vi "GFGTranslator.vi"(6 "boolean_ip":bool, 7 "Action":string, 8 "numeric_ip":dbl, 9 "string_ip":string="no. frames to acquire", 10 "GFG_var_name":string="no. frames to acquire", 11 "DataType":string) -> (0 "boolean_op":bool, 1 "numeric_op":dbl, 2 "string_op":string="no. frames to acquire", 3 "status":string, 4 "variant_op":variant, 5 "array_op":i16[][](array[numeric]))   [LabVIEW 2012]
doc: "SciScan 1.2 160622\nGFGTranslator 1.1 151001\n\nThis VI acts as an intermediate between a Python script and the LabVIEW SciScan application. Before using this VI make sure that the file path is correctly set to point to GFG_Core.ref file (situated in the SciScan project folder).\n\nAnother thing to note is that this VI should NOT be included in a project (i.e., needs to be run as a stand-alone VI), else could result in LabVIEW crashing"
uses:
  <vilib>/Utility/VariantDataType/Type.ctl
  <vilib>/vision/Image Controls.llb/IMAQ Image.ctl
  <vilib>/Utility/VariantDataType/VariantType.lvlib
  <vilib>/regexp/Match Regular Expression.xnode
panel:
  # "INPUTS"
  # "OUTPUTS"
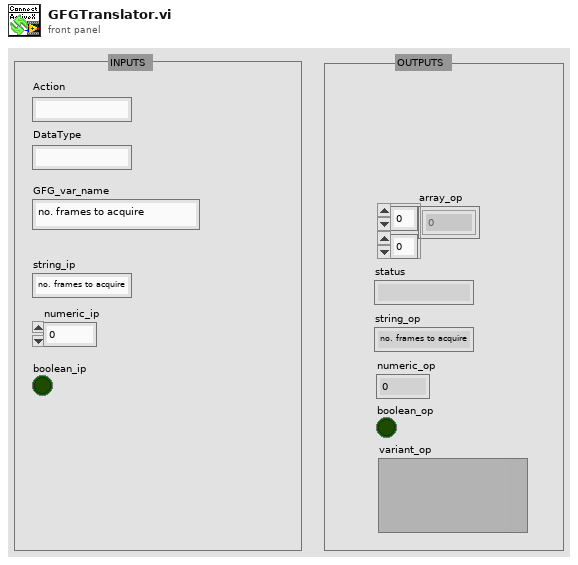
[diagram p1: front panel]
types:
  T1 = enum16{"open", "replace", "create", "open or create", "replace or create", "replace or create with confirmation"}
  T2 = typedef "VariantType.lvlib/Type.ctl" = enum8{"Invalid Type", "Void", "I8", "I16", "I32", "I64", "U8", "U16", "U32", "U64", "Single Float", "Double Float", "Extended Float", "Single Complex", "Double Complex", "Extended Complex", "Enum U8", "Enum U16", "Enum U32", "Enum U64", "Single Float With Unit", "Double Float With Unit", "Extended Float With Unit", "Single Complex with Unit", "Double Complex with Unit", "Extended Complex with Unit", "Boolean", "String", "Path", "Picture", "Tag", "Array", "Cluster", "Variant", "LV Variant", "Waveform", "Timestamp", "Digital Waveform", "Digital Data", "ExpressData", "Refnum", "External Data", "VI", "Poly VI", "LabVIEW Class Instance", "Fixed Point"}
  T3 = typedef "IMAQ Image.ctl" = refnum<image>
  T4 = cluster{"Channel 1 small":T3, "Channel 2 small":T3, "Channel 3 small":T3, "Channel 4 small":T3, "Channel 1 large":T3, "Channel 2 large":T3, "Channel 3 large":T3, "Channel 4 large":T3, "RGB overlay":T3, "ROI Image display":T3, "arb line scan display":T3, "Channel 5 large":T3}
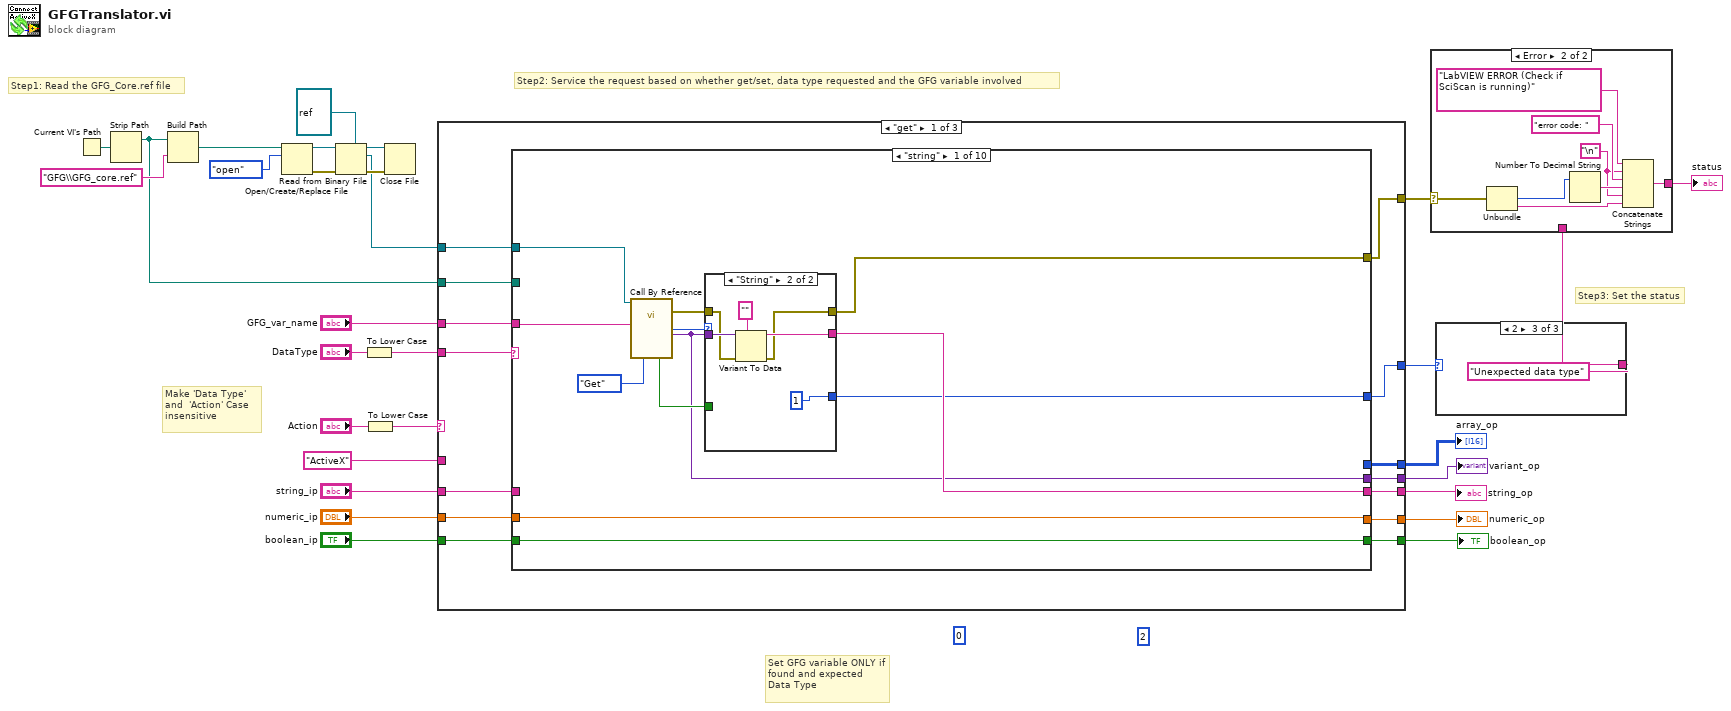
[diagram p0: block diagram]
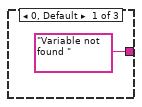
[diagram p3: hidden frame]
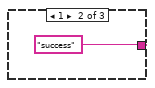
[diagram p4: hidden frame]
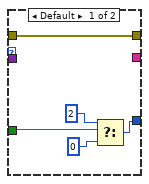
[diagram p5: hidden frame]
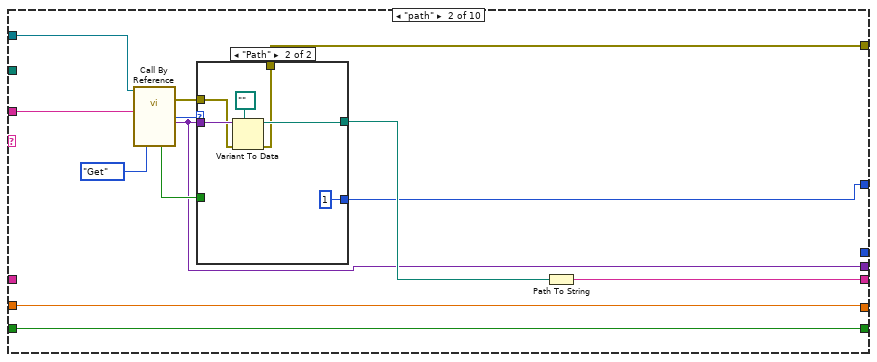
[diagram p6: hidden frame]
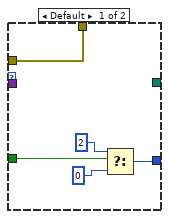
[diagram p7: hidden frame]
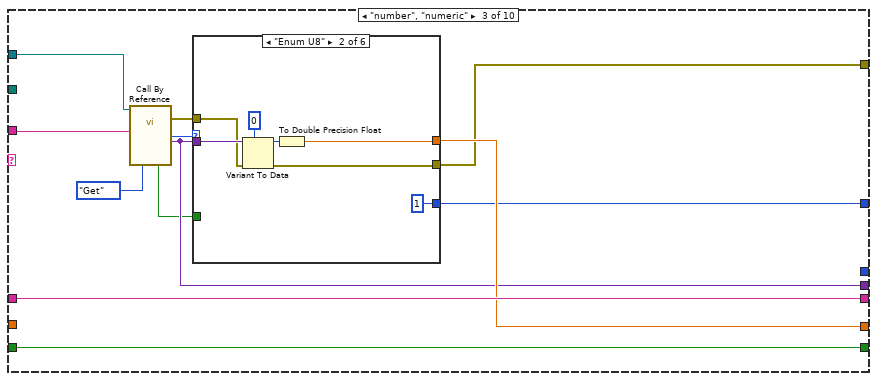
[diagram p8: hidden frame]
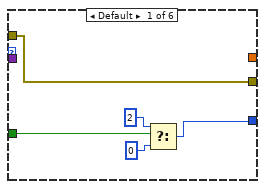
[diagram p9: hidden frame]
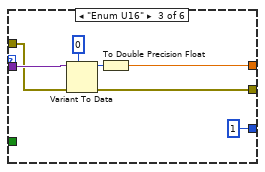
[diagram p10: hidden frame]
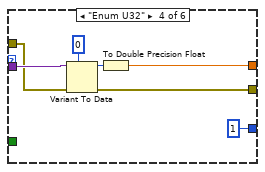
[diagram p11: hidden frame]
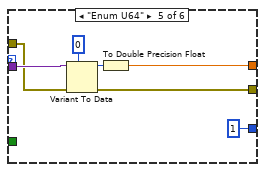
[diagram p12: hidden frame]
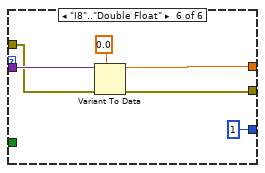
[diagram p13: hidden frame]
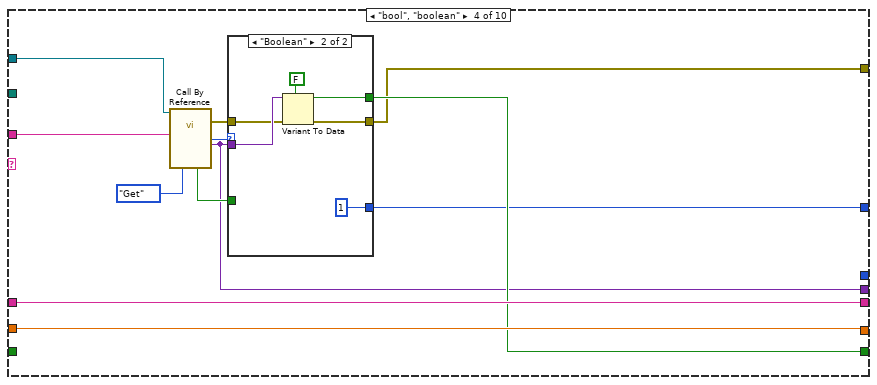
[diagram p14: hidden frame]
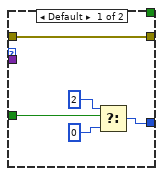
[diagram p15: hidden frame]
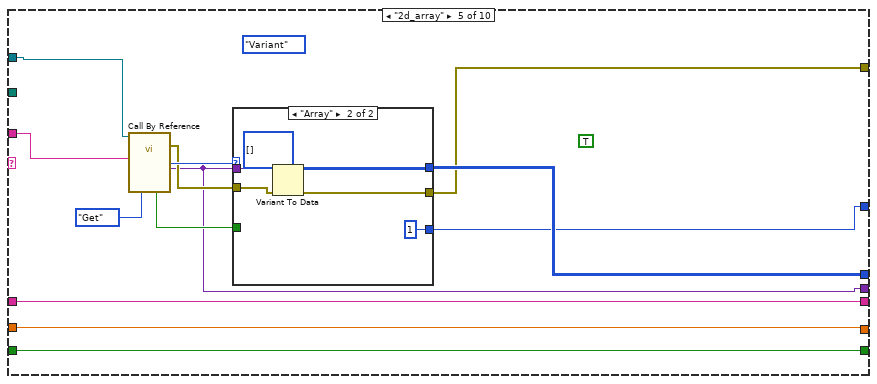
[diagram p16: hidden frame]
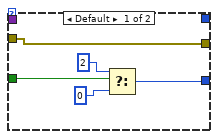
[diagram p17: hidden frame]
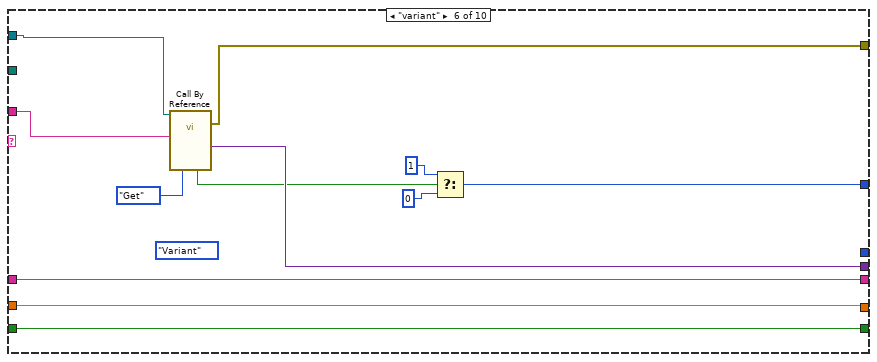
[diagram p18: hidden frame]
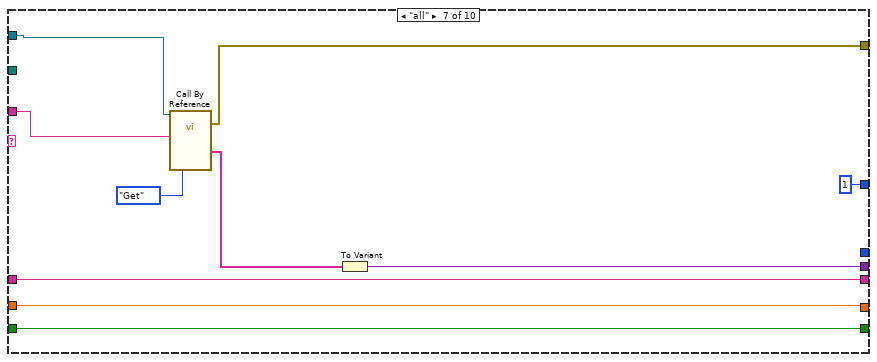
[diagram p19: hidden frame]
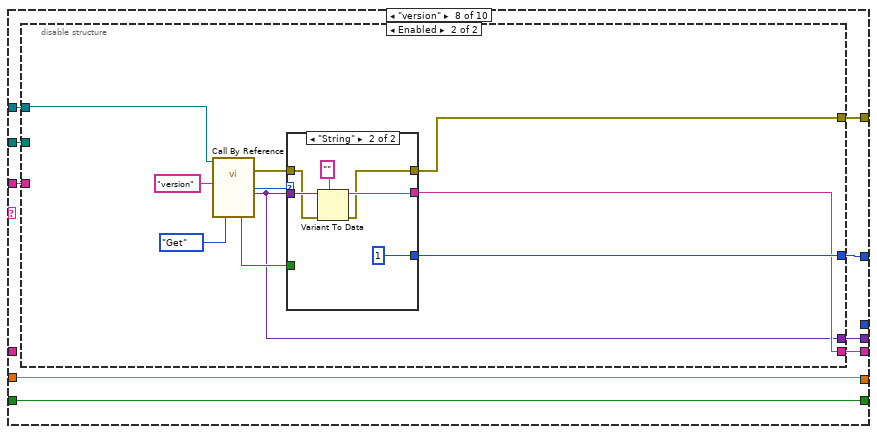
[diagram p20: hidden frame]
diagram:
  (unwired) 0
  (unwired) 2
  # "Set GFG variable ONLY if found and expected Data Type"
  # "Step3: Set the status"
  # "Step2: Service the request based on whether get/set, data type requested and the GFG variable involved"
  # "Step1: Read the GFG_Core.ref file"
  # "Make 'Data Type'\nand  'Action' Case\ninsensitive"
  n1 = Current VI's Path() -> (path=w10:path)
  n2 = Strip Path(path=w10) -> (stripped path=w7:path)  [unwired: 1 out]
  n3 = Build Path(base path=w7, name or relative path="GFG\\GFG_core.ref") -> (appended path=w8:path)
  n4 = Open/Create/Replace File(file path (use dialog)=w8, operation (0:open)=T1."open") -> (refnum out=w17:refnum<file>, error out=w18:errorcluster)  [unwired: 4 in, 1 out]
  n5 = Read from Binary File(5:refnum<vi> refnum ("type specifier VI Refnum (for type only)"), 8:w18, 11:w17) -> (0:w15:errorcluster, 2:w13:refnum<vi>, 3:w16:refnum<file>)  [unwired: 3 in, 1 out]
  n6 = To Lower Case(string="DataType") -> (all lower case string=w20:string)
  n7 = To Lower Case(string="Action") -> (all lower case string=w21:string)
  n8 = Close File(refnum=w16, error in=w15) -> ()  [unwired: 2 out]
  n9 = case shown="\"get\"" w21 {
    tunnel: w20 -> [w43 _ w578]
    tunnel: "GFG_var_name" -> [w42 _ w587]
    tunnel: [w41 w575 w585] -> w3
    tunnel: w13 -> [w40 _ w584]
    tunnel: "string_ip" -> [w38 w575 w586]
    tunnel: "ActiveX" ("Source VI") -> [_ _ w583]
    tunnel: "numeric_ip" -> [w37 w574 w582]
    tunnel: "boolean_ip" -> [w36 w573 w581]
    tunnel: [w39 w574 w580] -> w2
    tunnel: [w35 w573 w579] -> w22
    tunnel: [w34 _ _] -> w12
    tunnel: [w33 _ _] -> w11
    tunnel: w7 -> [w32 _ _]
    tunnel: [w31 errorcluster {"status"=TRUE, "code"=0, "source"="Undefined command received from ActiveX client"} ("error out") w577] -> w6
    tunnel: [w30 0 w576] -> w1
    frame "get" {
      n10 = case shown="\"string\"" w43 {
        tunnel: w42 -> [w51 w74 w98 w149 w173 w197 w207 w215 w527 _]
        tunnel: [w49 w79 w102 w152 w176 w199 w209 w216 w542 w570] -> w41
        tunnel: w40 -> [w50 w73 w97 w148 w172 w196 w204 w213 w537 _]
        tunnel: [w55 w78 w96 w153 w177 w200 w210 w219 w543 w569] -> w39
        tunnel: w38 -> [_ _ w102 w152 w176 w199 w209 _ w542 w570]
        tunnel: w37 -> [w55 w78 _ w153 w177 w200 w210 w219 w543 w569]
        tunnel: w36 -> [w54 w77 w101 _ w171 w195 w206 w218 w541 w568]
        tunnel: [w54 w77 w101 w147 w171 w195 w206 w218 w541 w568] -> w35
        tunnel: [_ _ _ _ w170 _ _ _ w540 _] -> w34
        tunnel: [w44 w67 w95 w142 w165 w194 w205 w211 w525 _] -> w33
        tunnel: w32 -> [_ _ _ _ _ _ _ w217 _ _]
        tunnel: [w47 w71 w94 w145 w168 w193 w203 w214 w529 errorcluster {"status"=TRUE, "code"=0, "source"="Undefined data Type"} ("error out")] -> w31
        tunnel: [w45 w68 w91 w143 w166 w189 1 w212 w528 2] -> w30
        frame "string" {
          n11 = call-by-ref "?"(reference=w50, "Variable Name in"=w51, "Action"=enum16{"Init", "Set", "Get"}."Get") -> (error out=w48:errorcluster, "Found/Replaced"=w46:bool, "Data Type Out"=w53:T2, "Variant Out"=w44:variant)  [unwired: 12 in, 5 out]
          n12 = case shown="\"String\"" w53 {
            tunnel: w44 -> [_ w66]
            tunnel: [_ w65] -> w49
            tunnel: w48 -> [w60 w63]
            tunnel: [w60 w62] -> w47
            tunnel: w46 -> [w58 _]
            tunnel: [w57 1] -> w45
            frame Default {
              n13 = Select(t=2, s=w58, f=0) -> (s? t:f=w57:i32)
            }
            frame "String" {
              n14 = Variant To Data(error in=w63, type="" ("string_ip"), Variant=w66) -> (data=w65:string, error out=w62:errorcluster)
            }
          }
        }
        frame "path" {
          n15 = call-by-ref "?"(reference=w73, "Variable Name in"=w74, "Action"=enum16{"Init", "Set", "Get"}."Get") -> (error out=w70:errorcluster, "Found/Replaced"=w69:bool, "Data Type Out"=w76:T2, "Variant Out"=w67:variant)  [unwired: 12 in, 5 out]
          n16 = case shown="\"Path\"" w76 {
            tunnel: w67 -> [_ w90]
            tunnel: [_ w89] -> w72
            tunnel: [w84 w87] -> w71
            tunnel: w70 -> [w84 w86]
            tunnel: w69 -> [w81 _]
            tunnel: [w80 1] -> w68
            frame Default {
              n17 = Select(t=2, s=w81, f=0) -> (s? t:f=w80:i32)
            }
            frame "Path" {
              n18 = Variant To Data(error in=w86, type=path "" ("Path"), Variant=w90) -> (data=w89:path, error out=w87:errorcluster)
            }
          }
          n19 = Path To String(path=w72) -> (string=w79:string)
        }
        frame "number", "numeric" {
          n20 = call-by-ref "?"(reference=w97, "Variable Name in"=w98, "Action"=enum16{"Init", "Set", "Get"}."Get") -> (error out=w93:errorcluster, "Found/Replaced"=w92:bool, "Data Type Out"=w100:T2, "Variant Out"=w95:variant)  [unwired: 12 in, 5 out]
          n21 = case shown="\"Enum U8\"" w100 {
            tunnel: w95 -> [_ w112 w119 w126 w133 w140]
            tunnel: [_ w111 w118 w125 w132 w139] -> w96
            tunnel: [w107 w109 w116 w123 w131 w138] -> w94
            tunnel: w93 -> [w107 w110 w117 w124 w130 w137]
            tunnel: w92 -> [w104 _ _ _ _ _]
            tunnel: [w103 1 1 1 1 1] -> w91
            frame Default {
              n22 = Select(t=2, s=w104, f=0) -> (s? t:f=w103:i32)
            }
            frame "Enum U8" {
              n23 = Variant To Data(error in=w110, type=u8 0 ("numeric_ip"), Variant=w112) -> (data=w113:u8, error out=w109:errorcluster)
              n24 = To Double Precision Float(number=w113) -> (double precision float=w111:dbl)
            }
            frame "Enum U16" {
              n25 = Variant To Data(error in=w117, type=u16 0 ("numeric_ip"), Variant=w119) -> (data=w120:u16, error out=w116:errorcluster)
              n26 = To Double Precision Float(number=w120) -> (double precision float=w118:dbl)
            }
            frame "Enum U32" {
              n27 = Variant To Data(error in=w124, type=u32 0 ("numeric_ip"), Variant=w126) -> (data=w127:u32, error out=w123:errorcluster)
              n28 = To Double Precision Float(number=w127) -> (double precision float=w125:dbl)
            }
            frame "Enum U64" {
              n29 = Variant To Data(error in=w130, type=u64 0 ("numeric_ip"), Variant=w133) -> (data=w134:u64, error out=w131:errorcluster)
              n30 = To Double Precision Float(number=w134) -> (double precision float=w132:dbl)
            }
            frame "I8".."Double Float" {
              n31 = Variant To Data(error in=w137, type=0.0 ("numeric_ip"), Variant=w140) -> (data=w139:dbl, error out=w138:errorcluster)
            }
          }
        }
        frame "bool", "boolean" {
          n32 = call-by-ref "?"(reference=w148, "Variable Name in"=w149, "Action"=enum16{"Init", "Set", "Get"}."Get") -> (error out=w146:errorcluster, "Found/Replaced"=w144:bool, "Data Type Out"=w151:T2, "Variant Out"=w142:variant)  [unwired: 12 in, 5 out]
          n33 = case shown="\"Boolean\"" w151 {
            tunnel: w142 -> [_ w164]
            tunnel: [_ w162] -> w147
            tunnel: w146 -> [w158 w161]
            tunnel: [w158 w160] -> w145
            tunnel: w144 -> [w157 _]
            tunnel: [w154 1] -> w143
            frame Default {
              n34 = Select(t=2, s=w157, f=0) -> (s? t:f=w154:i32)
            }
            frame "Boolean" {
              n35 = Variant To Data(error in=w161, type=FALSE, Variant=w164) -> (data=w162:bool, error out=w160:errorcluster)
            }
          }
        }
        frame "2d_array" {
          (unwired) TRUE ("Found/Replaced")
          (unwired) Type."Variant" ("Data Type Out")
          n36 = call-by-ref "?"(reference=w172, "Variable Name in"=w173, "Action"=enum16{"Init", "Set", "Get"}."Get") -> (error out=w169:errorcluster, "Found/Replaced"=w167:bool, "Data Type Out"=w175:T2, "Variant Out"=w165:variant)  [unwired: 12 in, 5 out]
          n37 = case shown="\"Array\"" w175 {
            tunnel: w165 -> [_ w188]
            tunnel: [_ w187] -> w170
            tunnel: w169 -> [w182 w185]
            tunnel: [w182 w184] -> w168
            tunnel: w167 -> [w179 _]
            tunnel: [w178 1] -> w166
            frame Default {
              n38 = Select(t=2, s=w179, f=0) -> (s? t:f=w178:i32)
            }
            frame "Array" {
              n39 = Variant To Data(error in=w185, type=i16[][] [], Variant=w188) -> (data=w187:i16[][], error out=w184:errorcluster)
            }
          }
        }
        frame "variant" {
          (unwired) Type."Variant" ("Data Type Out")
          n40 = call-by-ref "?"(reference=w196, "Variable Name in"=w197, "Action"=enum16{"Init", "Set", "Get"}."Get") -> (error out=w193:errorcluster, "Found/Replaced"=w190:bool, "Variant Out"=w194:variant)  [unwired: 12 in, 6 out]
          n41 = Select(t=1, s=w190, f=0) -> (s? t:f=w189:i32)
        }
        frame "all" {
          n42 = call-by-ref "?"(reference=w204, "Variable Name in"=w207, "Action"=enum16{"Init", "Set", "Get"}."Get") -> (error out=w203:errorcluster, "All Variable Names Out"=w202:string[])  [unwired: 12 in, 7 out]
          n43 = To Variant(anything=w202) -> (Variant=w205:variant)
        }
        frame "version" {
          n44 = disable-structure shown="Enabled" {
            disable-tunnel: w217 -> [w227 _]
            disable-tunnel: [w226 w505] -> w216
            disable-tunnel: w215 -> [w224 _]
            disable-tunnel: [w223 w507] -> w214
            disable-tunnel: w213 -> [w221 w509]
            disable-tunnel: [w220 w506] -> w212
            disable-tunnel: [_ w504] -> w211
            frame Disabled {
              n45 = To Lower Case(string=w224) -> (all lower case string=w228:string)
              n46 = xnode "Match Regular Expression"("input string"=w228, "regular expression"=".lvproj|.vi") -> ("before match"=w225:string, "error out"=w222:errorcluster)  [unwired: 4 in, 3 out]
              n47 = case shown="Default" w225 {
                selector: w225 -> [_ w357 _]
                tunnel: w227 -> [w344 _ _]
                tunnel: [w349 w362 w499] -> w226
                tunnel: [w348 w356 w497] -> w223
                tunnel: w222 -> [w347 w355 w496]
                tunnel: w221 -> [_ _ _]
                tunnel: [1 w354 1] -> w220
                frame "sci_scan", "sciscan" {
                  n48 = Build Path(base path=w344, name or relative path="Sci_Scan.lvproj") -> (appended path=w342:path)
                  n49 = invoke class="App" method="Project.Open"(error in=w347, "Path"=w342) -> (error out=w345:errorcluster, "Project:Open"=w346:refnum<vi>)  [unwired: 2 in, 2 out]
                  n50 = property class="Project"(reference=w346, error in=w345) -> (reference out=w352:refnum<vi>, error out=w353:errorcluster, "Description"=w351:string)
                  n51 = Close Reference(reference=w352, error in (no error)=w353) -> (error out=w348:errorcluster)
                  n52 = Match Pattern(string=w351, regular expression="[\\n,\\r]") -> (before substring=w349:string)  [unwired: 1 in, 3 out]
                }
                frame Default {
                  n53 = call "get all VIs in SciScan directory.vi"() -> ("All Files in Dir"=w358:path[])  [unwired: 11 in]
                  n54 = for {
                    tunnel: w358 -> [w367] mode=indexing
                    tunnel: [w364] -> w359 mode=indexing
                    n55 = Strip Path(path=w367) -> (name=w365:string)  [unwired: 1 out]
                    n56 = To Lower Case(string=w365) -> (all lower case string=w366:string)
                    n57 = xnode "Match Regular Expression"("input string"=w366, "regular expression"=".lvproj|.vi") -> ("before match"=w364:string)  [unwired: 4 in, 4 out]
                  }
                  n58 = Search 1D Array(1D array=w359, element=w357) -> (index of element=w361:i32)  [unwired: 1 in]
                  n59 = Greater Or Equal To 0?(x=w361) -> (x >= 0?=w360:bool)
                  n60 = case shown="False" w360 {
                    tunnel: ["The specified project/VI name not found" ("Description") w493] -> w362
                    tunnel: w361 -> [_ w490]
                    tunnel: w358 -> [_ w486]
                    tunnel: [w480 w485] -> w356
                    tunnel: w355 -> [w480 w484]
                    tunnel: [0 1] -> w354
                    frame False {
                    }
                    frame True {
                      n61 = Index Array(array=w486, index=w490) -> (element=w489:path)
                      n62 = Open VI Reference(vi path=w489, error in (no error)=w484) -> (vi reference=w492:refnum<vi>, error out=w483:errorcluster)  [unwired: 4 in]
                      n63 = property class="VI"(reference=w492, error in=w483) -> (reference out=w487:refnum<vi>, error out=w488:errorcluster, "Description"=w491:string)
                      n64 = Match Pattern(string=w491, regular expression="[\\n,\\r]") -> (before substring=w493:string)  [unwired: 1 in, 3 out]
                      n65 = Close Reference(reference=w487, error in (no error)=w488) -> (error out=w485:errorcluster)
                    }
                  }
                }
                frame "gfgtranslator" {
                  n66 = control-ref of="This VI"() -> (w498:refnum<vi>)
                  n67 = property class="VI"(reference=w498, error in=w496) -> (reference out=w502:refnum<vi>, error out=w503:errorcluster, "Description"=w501:string)
                  n68 = Close Reference(reference=w502, error in (no error)=w503) -> (error out=w497:errorcluster)
                  n69 = Match Pattern(string=w501, regular expression="[\\n,\\r]") -> (before substring=w499:string)  [unwired: 1 in, 3 out]
                }
              }
            }
            frame Enabled {
              n70 = call-by-ref "?"(reference=w509, "Variable Name in"="version", "Action"=enum16{"Init", "Set", "Get"}."Get") -> (error out=w511:errorcluster, "Found/Replaced"=w510:bool, "Data Type Out"=w513:T2, "Variant Out"=w504:variant)  [unwired: 12 in, 5 out]
              n71 = case shown="\"String\"" w513 {
                tunnel: w504 -> [_ w524]
                tunnel: [_ w523] -> w505
                tunnel: w511 -> [w518 w521]
                tunnel: [w518 w520] -> w507
                tunnel: w510 -> [w516 _]
                tunnel: [w515 1] -> w506
                frame Default {
                  n72 = Select(t=2, s=w516, f=0) -> (s? t:f=w515:i32)
                }
                frame "String" {
                  n73 = Variant To Data(error in=w521, type="" ("string_ip"), Variant=w524) -> (data=w523:string, error out=w520:errorcluster)
                }
              }
            }
          }
        }
        frame "image" {
          w535 = T4 {"Channel 1 small"=refnum, "Channel 2 small"=refnum, "Channel 3 small"=refnum, "Channel 4 small"=refnum, "Channel 1 large"=refnum, "Channel 2 large"=refnum, "Channel 3 large"=refnum, "Channel 4 large"=refnum, "RGB overlay"=refnum, "ROI Image display"=refnum, "arb line scan display"=refnum, "Channel 5 large"=refnum}  # output cluster
          n74 = call-by-ref "?"(reference=w537, "Variable Name in"="ImageRefCluster", "Action"=enum16{"Init", "Set", "Get"}."Get") -> (reference out=w526:refnum<vi>, error out=w530:errorcluster, "Variant Out"=w525:variant)  [unwired: 12 in, 6 out]
          n75 = Variant To Data(error in=w530, type=w535, Variant=w525) -> (data=w534:T4, error out=w533:errorcluster)
          n76 = Cluster To Array(cluster=w534) -> (array=w536:T3[])
          n77 = case shown="No Error" w533 {
            selector: w533 -> [w546 w555]
            tunnel: w536 -> [w549 _]
            tunnel: w527 -> [w548 _]
            tunnel: [w547 _] -> w531
            tunnel: [w545 _] -> w532
            tunnel: [w544 w555] -> w529
            frame No Error {
              n78 = for {
                tunnel: w549 -> [w550] mode=indexing
                tunnel: w548 -> [w553]
                tunnel: [w552] -> w547
                tunnel: [w550] -> w545
                tunnel: w546 -> [_]
                tunnel: [w551] -> w544
                stop <- w552 stop-if-true
                n79 = call "IMAQ GetImageInfo"("Image"=w550) -> ("error out"=w551:errorcluster, "Image Name"=w554:string)  [unwired: 3 in, 6 out]
                n80 = Equal?(x=w554, y=w553) -> (x = y?=w552:bool)
              }
            }
            frame Error {
            }
          }
          n81 = case shown="False" w531 {
            tunnel: [_ w565] -> w540
            tunnel: w532 -> [_ w564]
            tunnel: [w556 1] -> w528
            tunnel: w527 -> [w561 _]
            tunnel: w526 -> [w560 _]
            frame False {
              # "The variable has not been found in the ImageRefCluster.\nCheck if the variable is present in the GFG and report error accordingly"
              n82 = call-by-ref "?"(reference=w560, "Variable Name in"=w561, "Action"=enum16{"Init", "Set", "Get"}."Get") -> ("Found/Replaced"=w557:bool)  [unwired: 12 in, 8 out]
              n83 = Select(t=2, s=w557, f=0) -> (s? t:f=w556:i32)
            }
            frame True {
              n84 = call "IMAQ ImageToArray"("Image"=w564) -> ("Image Pixels (I16)"=w565:i16[][])  [unwired: 3 in, 4 out]
            }
          }
        }
        frame Default {
        }
      }
    }
    frame Default {
    }
    frame "set" {
      n85 = case shown="\"booleanref\"" w578 {
        tunnel: w587 -> [w592 w641 w673 w718 w752 _]
        tunnel: w586 -> [w600 w648 w680 w725 w765 w804]
        tunnel: [w600 w648 w680 w725 w765 w804] -> w585
        tunnel: w584 -> [w596 w643 w676 w721 w751 _]
        tunnel: w583 -> [w599 _ w668 w726 _ _]
        tunnel: w582 -> [w598 w645 w679 w723 w764 w805]
        tunnel: w581 -> [w597 w646 w678 w724 w750 w806]
        tunnel: [w598 w645 w679 w723 w764 w805] -> w580
        tunnel: [w597 w646 w678 w724 w750 w806] -> w579
        tunnel: [w591 w638 w671 w716 w749 errorcluster {"status"=TRUE, "code"=0, "source"="Undefined data type received from ActiveX client"} ("error out")] -> w577
        tunnel: [w588 w636 w669 w714 w747 2 ("f")] -> w576
        frame "string" {
          # "Check if GFG variable exists"
          # "Set GFG variable ONLY if found and expected Data Type"
          n86 = call-by-ref "?"(reference=w596, "Variable Name in"=w592, "Action"=enum16{"Init", "Set", "Get", "Clear"}."Get") -> (reference out=w595:refnum<vi>, error out=w594:errorcluster, "Found/Replaced"=w590:bool, "Data Type Out"=w589:T2)  [unwired: 12 in, 5 out]
          n87 = case shown="True" w590 {
            tunnel: w600 -> [w604 w625]
            tunnel: w599 -> [w602 w624]
            tunnel: w595 -> [w603 w623]
            tunnel: w594 -> [w605 w622]
            tunnel: w592 -> [w606 w621]
            tunnel: [w601 w620] -> w591
            tunnel: w589 -> [_ w619]
            tunnel: [w607 w618] -> w588
            frame False {
              n88 = case shown="\"SetAbsXYZ\", \"SetVirtXYZ\"" w606 {
                selector: w606 -> [_ w615]
                tunnel: [0 1] -> w607
                tunnel: w605 -> [w608 w612]
                tunnel: w604 -> [_ w614]
                tunnel: w603 -> [_ w611]
                tunnel: w602 -> [_ w613]
                tunnel: [w608 w610] -> w601
                frame Default {
                }
                frame "SetAbsXYZ", "SetVirtXYZ" {
                  n89 = call-by-ref "?"(reference=w611, error in=w612, "Variable Name in"=w615, "Variant in"=w614, "Source VI"=w613, "Action"=enum16{"Init", "Set", "Get", "Clear"}."Set") -> (error out=w610:errorcluster)  [unwired: 9 in, 8 out]
                }
              }
            }
            frame True {
              n90 = case shown="\"String\"" w619 {
                tunnel: w625 -> [_ w635]
                tunnel: w624 -> [_ w634]
                tunnel: w623 -> [_ w633]
                tunnel: w622 -> [w627 w632]
                tunnel: w621 -> [_ w631]
                tunnel: [w627 w630] -> w620
                tunnel: [2 1] -> w618
                frame Default {
                }
                frame "String" {
                  n91 = call-by-ref "?"(reference=w633, error in=w632, "Variable Name in"=w631, "Variant in"=w635, "Source VI"=w634, "Action"=enum16{"Init", "Set", "Get", "Clear"}."Set") -> (error out=w630:errorcluster)  [unwired: 9 in, 8 out]
                }
              }
            }
          }
        }
        frame "path" {
          # "Set GFG variable ONLY if found and expected Data Type"
          # "Check if GFG variable exists"
          n92 = call-by-ref "?"(reference=w643, "Variable Name in"=w641, "Action"=enum16{"Init", "Set", "Get", "Clear"}."Get") -> (reference out=w642:refnum<vi>, error out=w639:errorcluster, "Found/Replaced"=w640:bool, "Data Type Out"=w637:T2)  [unwired: 12 in, 5 out]
          n93 = String To Path(string=w648) -> (path=w647:path)
          n94 = case shown="True" w640 {
            selector: w640 -> [_ w653]
            tunnel: w647 -> [_ w658]
            tunnel: w642 -> [_ w657]
            tunnel: w641 -> [_ w656]
            tunnel: w639 -> [w650 w655]
            tunnel: [w650 w654] -> w638
            tunnel: w637 -> [_ w652]
            tunnel: [0 w651] -> w636
            frame False {
            }
            frame True {
              n95 = case shown="\"Path\"" w652 {
                tunnel: w658 -> [_ w667]
                tunnel: w657 -> [_ w666]
                tunnel: w656 -> [_ w665]
                tunnel: w655 -> [w660 w664]
                tunnel: [w660 w663] -> w654
                tunnel: w653 -> [_ _]
                tunnel: [2 1] -> w651
                frame Default {
                }
                frame "Path" {
                  n96 = call-by-ref "?"(reference=w666, error in=w664, "Variable Name in"=w665, "Variant in"=w667, "Action"=enum16{"Init", "Set", "Get", "Clear"}."Set") -> (error out=w663:errorcluster)  [unwired: 10 in, 8 out]
                }
              }
            }
          }
        }
        frame "number", "numeric" {
          # "Set GFG variable ONLY if found and expected Data Type"
          # "Check if GFG variable exists"
          n97 = call-by-ref "?"(reference=w676, "Variable Name in"=w673, "Action"=enum16{"Init", "Set", "Get", "Clear"}."Get") -> (reference out=w675:refnum<vi>, error out=w674:errorcluster, "Found/Replaced"=w672:bool, "Data Type Out"=w670:T2)  [unwired: 12 in, 5 out]
          n98 = case shown="False" w672 {
            tunnel: w679 -> [w684 w704]
            tunnel: w675 -> [w686 w703]
            tunnel: w674 -> [w685 w702]
            tunnel: w673 -> [w681 w701]
            tunnel: [w682 w700] -> w671
            tunnel: w670 -> [_ w699]
            tunnel: [w687 w698] -> w669
            tunnel: w668 -> [w683 _]
            frame False {
              n99 = case shown="\"absX\", \"absY\", \"absZ\"" w681 {
                selector: w681 -> [_ w693]
                tunnel: [0 1] -> w687
                tunnel: w686 -> [_ w695]
                tunnel: w685 -> [w689 w694]
                tunnel: w684 -> [_ w692]
                tunnel: w683 -> [_ w691]
                tunnel: [w689 w690] -> w682
                frame "False", Default {
                }
                frame "absX", "absY", "absZ" {
                  n100 = call-by-ref "?"(reference=w695, error in=w694, "Variable Name in"=w693, "Variant in"=w692, "Source VI"=w691, "Action"=enum16{"Init", "Set", "Get", "Clear"}."Set") -> (error out=w690:errorcluster)  [unwired: 9 in, 8 out]
                }
              }
            }
            frame True {
              n101 = case shown="\"I8\"..\"Double Float\", \"Enum U8\"..\"Enum U64\"" w699 {
                tunnel: w704 -> [_ w713]
                tunnel: w703 -> [_ w712]
                tunnel: w702 -> [w705 w711]
                tunnel: w701 -> [_ w710]
                tunnel: [w705 w709] -> w700
                tunnel: [2 1] -> w698
                frame Default {
                }
                frame "I8".."Double Float", "Enum U8".."Enum U64" {
                  n102 = call-by-ref "?"(reference=w712, error in=w711, "Variable Name in"=w710, "Variant in"=w713, "Action"=enum16{"Init", "Set", "Get", "Clear"}."Set") -> (error out=w709:errorcluster)  [unwired: 10 in, 8 out]
                }
              }
            }
          }
        }
        frame "bool", "boolean" {
          # "Set GFG variable ONLY if found and expected Data Type"
          # "Check if GFG variable exists"
          n103 = call-by-ref "?"(reference=w721, "Variable Name in"=w718, "Action"=enum16{"Init", "Set", "Get", "Clear"}."Get") -> (reference out=w720:refnum<vi>, error out=w719:errorcluster, "Found/Replaced"=w717:bool, "Data Type Out"=w715:T2)  [unwired: 12 in, 5 out]
          n104 = case shown="False" w717 {
            tunnel: w726 -> [_ w736]
            tunnel: w724 -> [_ w735]
            tunnel: w720 -> [_ w734]
            tunnel: w719 -> [w728 w733]
            tunnel: w718 -> [_ w732]
            tunnel: [w728 w731] -> w716
            tunnel: w715 -> [_ w730]
            tunnel: [0 w729] -> w714
            frame False {
            }
            frame True {
              n105 = case shown="\"Boolean\"" w730 {
                tunnel: w736 -> [_ w746]
                tunnel: w735 -> [_ w745]
                tunnel: w734 -> [_ w744]
                tunnel: w733 -> [w738 w743]
                tunnel: w732 -> [_ w742]
                tunnel: [w738 w741] -> w731
                tunnel: [2 1] -> w729
                frame Default {
                }
                frame "Boolean" {
                  n106 = call-by-ref "?"(reference=w744, error in=w743, "Variable Name in"=w742, "Variant in"=w745, "Source VI"=w746, "Action"=enum16{"Init", "Set", "Get", "Clear"}."Set") -> (error out=w741:errorcluster)  [unwired: 9 in, 8 out]
                }
              }
            }
          }
        }
        frame "booleanref" {
          w757 = ".CtrlRef" ("string")
          # "Add a .CtrlRef"
          # "Set the Control ONLY if found, and the reference type is a 'Boolean Refnum'"
          # "Check if GFG variable exists"
          n107 = Search and Replace String(replace all?=TRUE ("replace all? (F)"), input string=w752, search string="[\\t \\r \\n \\s]+", replace string="." ("replace string (\"\")")) -> (result string=w756:string)  [unwired: 4 in, 3 out]
          n108 = Match Pattern(string=w756, regular expression=w757) -> (offset past match=w758:i32)  [unwired: 1 in, 3 out]
          n109 = case shown="-1" w758 {
            tunnel: [w798 w801] -> w760
            tunnel: w756 -> [w798 w800]
            tunnel: w757 -> [_ w799]
            frame 0, Default {
            }
            frame -1 {
              n110 = Concatenate Strings(w800, w799) -> (w801:string)
            }
          }
          n111 = call-by-ref "?"(reference=w751, "Variable Name in"=w760, "Action"=enum16{"Init", "Set", "Get"}."Get") -> (error out=w748:errorcluster, "Found/Replaced"=w762:bool, "Data Type Out"=w761:T2, "Variant Out"=w763:variant)  [unwired: 12 in, 5 out]
          n112 = case shown="\"Refnum\"" w761 {
            tunnel: w762 -> [_ w770]
            tunnel: w763 -> [_ w773]
            tunnel: w750 -> [_ w772]
            tunnel: [w767 w771] -> w749
            tunnel: w748 -> [w767 w768]
            tunnel: [2 ("f") w769] -> w747
            frame Default {
            }
            frame "Refnum" {
              n113 = case shown="True" w770 {
                tunnel: w773 -> [_ w784]
                tunnel: [0 w776] -> w769
                tunnel: w772 -> [_ w778]
                tunnel: [w774 w777] -> w771
                tunnel: w768 -> [w774 _]
                frame False {
                }
                frame True {
                  w785 = refnum<vi> refnum  # Generic
                  n114 = Variant To Data(type=w785, Variant=w784) -> (data=w783:refnum<vi>, error out=w782:errorcluster)  [unwired: 1 in]
                  n115 = property class="Gen"(reference=w783, error in=w782) -> (reference out=w780:refnum<vi>, error out=w779:errorcluster, "ClassName"=w781:string)
                  n116 = case shown="\"Boolean\"" w781 {
                    tunnel: w780 -> [_ w796]
                    tunnel: w779 -> [w787 w795]
                    tunnel: w778 -> [_ w792]
                    tunnel: [w787 w789] -> w777
                    tunnel: [2 ("f") 1 ("f")] -> w776
                    frame "False", Default {
                    }
                    frame "Boolean" {
                      w797 = refnum<vi> refnum  # Boolean
                      n117 = To More Specific Class(target class=w797, reference=w796, error in=w795) -> (specific class reference=w794:refnum<vi>, error out=w793:errorcluster)
                      n118 = property class="Bool"(reference=w794, error in=w793, "Val(Sgnl)"=w792) -> (reference out=w790:refnum<vi>, error out=w791:errorcluster)
                      n119 = Close Reference(reference=w790, error in (no error)=w791) -> (error out=w789:errorcluster)
                    }
                  }
                }
              }
            }
          }
        }
        frame Default {
        }
      }
    }
  }
  "numeric_op" <- w2
  "boolean_op" <- w22
  "string_op" <- w3
  "array_op" <- w12
  "variant_op" <- w11
  n120 = case shown="2" w1 {
    tunnel: ["Variable not found " ("string_ip") "success" ("string_ip") "Unexpected data type" ("string_ip")] -> w4
    frame 0, Default {
    }
    frame 1 {
    }
    frame 2 {
    }
  }
  n121 = case shown="Error" w6 {
    selector: w6 -> [_ w818]
    tunnel: [w810 w816] -> w5
    tunnel: w4 -> [w810 _]
    frame No Error {
    }
    frame Error {
      w811 = "\n"
      n122 = Unbundle(w818) -> ("code"=w815:i32, "source"=w817:string)  [unwired: 1 out]
      n123 = Number To Decimal String(number=w815) -> (decimal integer string=w814:string)  [unwired: 1 in]
      n124 = Concatenate Strings("LabVIEW ERROR (Check if SciScan is running)" ("string"), w811, "error code: " ("string"), w814, w811, w817) -> (w816:string)
    }
  }
  "status" <- w5
